vi "Set Enable Heater Button Ref.vi"(8 "error in (no error)":errorcluster, 10 "Enable Heater Button Ref":refnum<vi>, 11 "Thermal Chamber Controller In":refnum<class "Thermal Chamber Controller.lvclass">) -> (0 "error out":errorcluster, 3 "Thermal Chamber Controller Out":refnum<class "Thermal Chamber Controller.lvclass">)   [LabVIEW 2020, in "Thermal Chamber Controller.lvclass"]
uses:
  Thermal Chamber Controller.lvclass
  <vilib>/Asteme/Triarc Framework/Process/Process.lvclass
  C:/Program Files (x86)/National Instruments/LabVIEW 2020/vi.lib/Asteme/Triarc Framework/View/View.lvclass
  C:/Program Files (x86)/National Instruments/LabVIEW 2020/vi.lib/Asteme/Triarc Framework/Process/Process.lvclass
  C:/Program Files (x86)/National Instruments/LabVIEW 2020/vi.lib/Asteme/Triarc Framework/Base/Base.lvclass
  C:/Program Files (x86)/National Instruments/LabVIEW 2020/vi.lib/Asteme/Triarc Framework/Error Handler Interface/Error Handler Interface.lvclass
  C:/Program Files (x86)/National Instruments/LabVIEW 2020/vi.lib/Asteme/Triarc Framework/Logging/Logging.lvclass
  C:/Users/anton/Documents/GitHub/Triarc-Examples/Thermal Chamber/Thermal Chamber Controller/Thermal Chamber Controller.lvclass
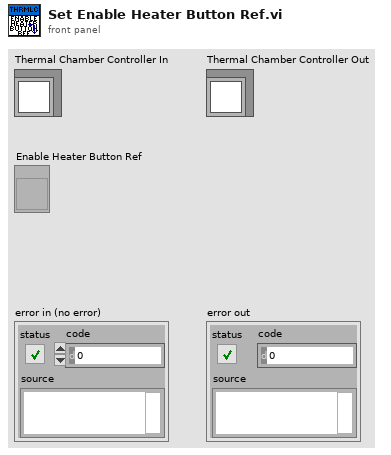
[diagram p1: front panel]
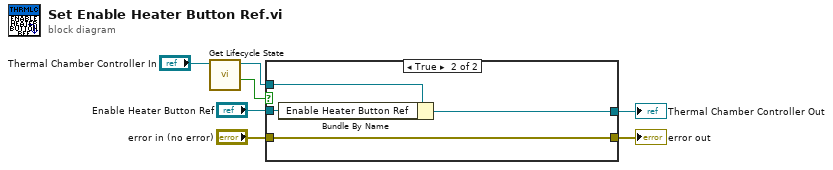
[diagram p0: block diagram]
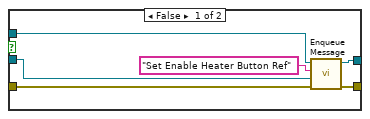
[diagram p2: hidden frame]
diagram:
  n1 = call <vilib>:"Get Lifecycle State.vi"("Process In"="Thermal Chamber Controller In") -> ("In Process Loop?"=w3:bool, "Process Out"=w6:refnum<class "Thermal Chamber Controller.lvclass">)  [unwired: 7 in, 2 out]
  n2 = case shown="True" w3 {
    tunnel: w6 -> [w13 w17]
    tunnel: [w12 w15] -> w5
    tunnel: "error in (no error)" -> [w8 w16]
    tunnel: [w9 w16] -> w4
    tunnel: "Enable Heater Button Ref" -> [w11 w14]
    frame False {
      n3 = call <vilib>:"Enqueue Message.vi"("error in (no error)"=w8, "Message Data"=w11, "Message"="Set Enable Heater Button Ref" ("API Message"), "Process In"=w13) -> ("error out"=w9:errorcluster, "Process Out"=w12:refnum<class "Thermal Chamber Controller.lvclass">)  [unwired: 6 in]
    }
    frame True {
      n4 = Bundle By Name(cluster=w17, "Enable Heater Button Ref"=w14) -> (w15:refnum<class "Thermal Chamber Controller.lvclass">)
    }
  }
  "error out" <- w4
  "Thermal Chamber Controller Out" <- w5
